vi "Envelope(SubVI).vi"(1 "x":dbl[](array[numeric])) -> (0 "Y":dbl[](array[numeric]))   [LabVIEW 2017]
uses:
  <vilib>/Analysis/NI_AALPro.lvlib
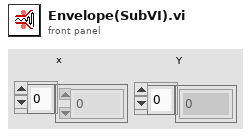
[diagram p1: front panel]
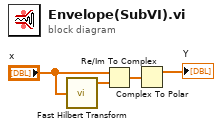
[diagram p0: block diagram]
diagram:
  n1 = call <vilib>:"Fast Hilbert Transform.vi"("X"="x") -> ("Hilbert{X}"=w4:dbl[])  [unwired: 1 out]
  n2 = Re/Im To Complex(1:w4, 2:"x") -> (0:w3:cdb[])
  n3 = Complex To Polar(r * e^(i*theta)=w3) -> (r=→"Y":dbl[])  [unwired: 1 out]
